vi "update stimulator ring entries (sub-vi).vi"(8 "error in (no error)":errorcluster, 9 "reset ring value? (F)":bool, 10 "ragged ring entry []":T1, 11 "port-odor ring refnum []":refnum<vi>[](array[refnum])) -> (0 "error out":errorcluster, 3 "port odor ring refnum [] out":refnum<vi>[](array[refnum]))   [LabVIEW 2021]
uses:
  type-defs/ragged ring entry 2D array cluster (typed def).ctl
  type-defs/ring string and value cluster (type def).ctl
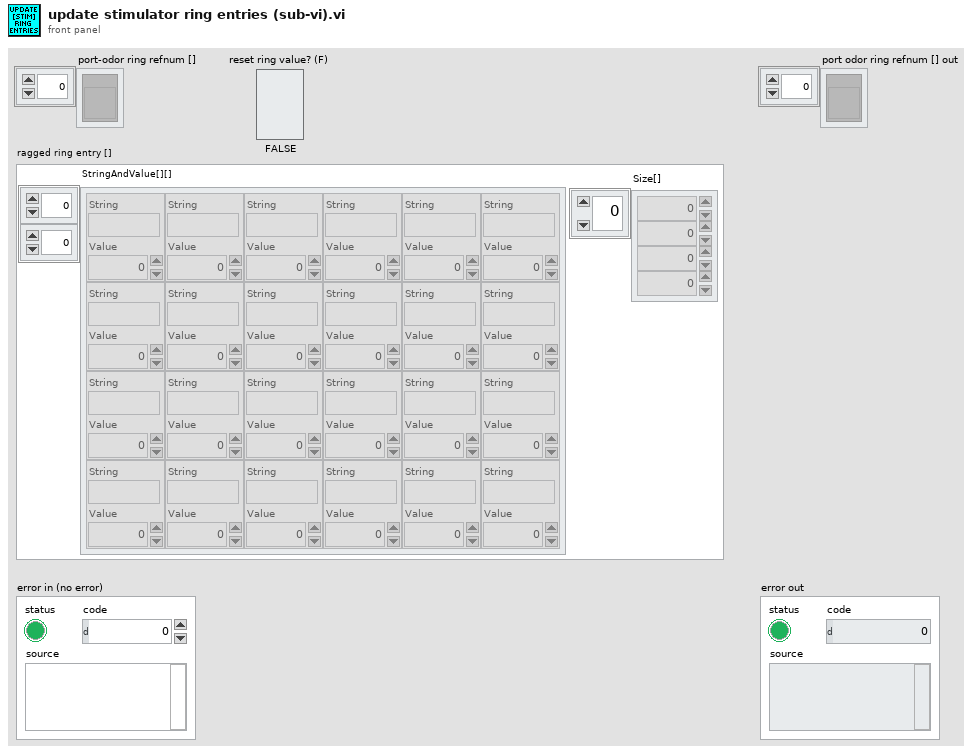
[diagram p1: front panel]
types:
  T1 = typedef "ragged ring entry 2D array cluster (typed def).ctl" = cluster{"StringAndValue[][]":T2[][], "Size[]":i32[]}
  T2 = typedef "ring string and value cluster (type def).ctl" = cluster{"String":string, "Value":u16}
  T3 = typedef "LVStringsAndValuesArrayTypeDef_U16.ctl" = cluster{"String":string, "Value":u16}[]
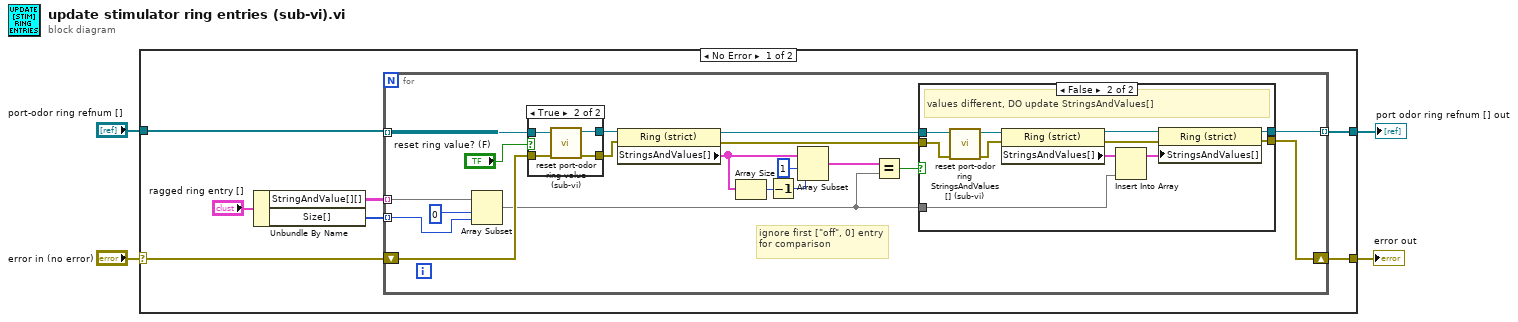
[diagram p0: block diagram]
diagram:
  n1 = case shown="No Error" "error in (no error)" {
    selector: "error in (no error)" -> [w11 w50]
    tunnel: [w10 w50] -> w3
    tunnel: "port-odor ring refnum []" -> [w9 w51]
    tunnel: [w8 w51] -> w1
    frame No Error {
      n2 = Unbundle By Name("ragged ring entry []") -> ("StringAndValue[][]"=w6:T2[][], "Size[]"=w5:i32[])
      n3 = for {
        shift-right: [w30] -> w10
        shift-left: w11 -> [w24]
        tunnel: w9 -> [w25] mode=indexing
        tunnel: [w29] -> w8 mode=indexing
        tunnel: w6 -> [w28] mode=indexing
        tunnel: w5 -> [w26] mode=indexing
        # "ignore first [\"off\", 0] entry\nfor comparison"
        n4 = Array Subset(array=w28, index=0, length=w26) -> (w13:T2[])
        n5 = case shown="True" "reset ring value? (F)" {
          tunnel: w25 -> [w44 w49]
          tunnel: [w44 w48] -> w22
          tunnel: [w45 w47] -> w20
          tunnel: w24 -> [w45 w46]
          frame False {
          }
          frame True {
            n6 = call "reset port-odor ring value (sub-vi).vi"("error in (no error)"=w46, "port-odor ring refnum"=w49) -> ("error out"=w47:errorcluster, "port-odor ring refnum out"=w48:refnum<vi>)  [unwired: 8 in]
          }
        }
        n7 = property class="Ring (strict)"(reference=w22, error in=w20) -> (reference out=w21:refnum<vi>, error out=w19:errorcluster, "StringsAndValues[]"=w17:T3)
        n8 = Array Size(array=w17) -> (size(s)=w16:i32)
        n9 = Decrement(x=w16) -> (x-1=w15:i32)
        n10 = Array Subset(array=w17, index=1, length=w15) -> (w14:T3)
        n11 = Equal?(x=w14, y=w13) -> (x = y?=w12:bool)
        n12 = case shown="False" w12 {
          tunnel: [w32 w37] -> w30
          tunnel: [w31 w36] -> w29
          tunnel: w21 -> [w31 w35]
          tunnel: w19 -> [w32 w34]
          tunnel: w13 -> [_ w33]
          frame True {
            # "values identical, do NOT update"
          }
          frame False {
            # "values different, DO update StringsAndValues[]"
            n13 = call "reset port-odor ring StringsAndValues[] (sub-vi).vi"("error in (no error)"=w34, "port-odor ring refnum"=w35) -> ("error out"=w39:errorcluster, "port-odor ring refnum out"=w40:refnum<vi>)  [unwired: 8 in]
            n14 = property class="Ring (strict)"(reference=w40, error in=w39) -> (reference out=w41:refnum<vi>, error out=w38:errorcluster, "StringsAndValues[]"=w43:T3)
            n15 = Insert Into Array(array=w43, new element=w33) -> (w42:T3)  [unwired: 1 in]
            n16 = property class="Ring (strict)"(reference=w41, error in=w38, "StringsAndValues[]"=w42) -> (reference out=w36:refnum<vi>, error out=w37:errorcluster)
          }
        }
      }
    }
    frame Error {
    }
  }
  "error out" <- w3
  "port odor ring refnum [] out" <- w1
